vi "1.7A_Test.vi"(3 "error in":errorcluster) -> (10 "error out":errorcluster)   [LabVIEW 2015]
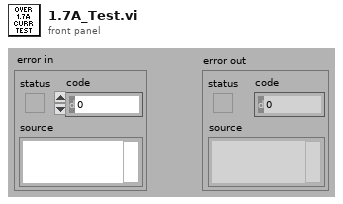
[diagram p1: front panel]
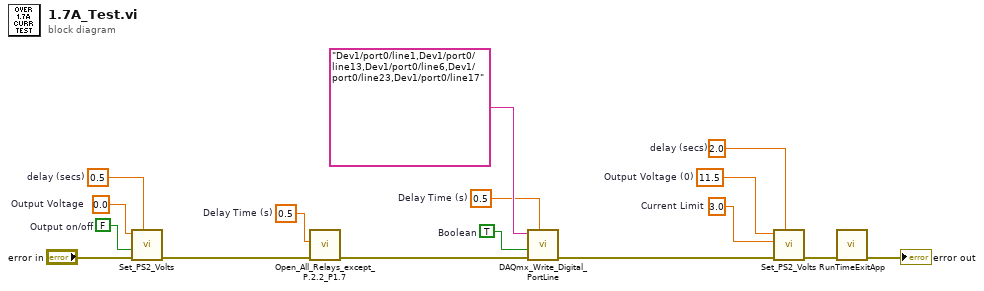
[diagram p0: block diagram]
diagram:
  w1 = 3.0  # Current Limit
  w2 = 0.5  # Delay Time (s)
  w3 = 0.5  # Delay Time (s)
  w6 = 0.0  # Output Voltage
  w7 = 0.5  # delay (secs)
  w8 = FALSE  # Output on/off
  w10 = 2.0  # delay (secs)
  w14 = 11.5  # Output Voltage (0)
  w16 = TRUE  # Boolean
  n1 = call "Set_PS2_Volts.vi"("delay (secs)"=w7, "error in"="error in", "Output on/off"=w8, "Output Voltage"=w6) -> ("error out"=w4:errorcluster)  [unwired: 5 in, 2 out]
  n2 = call "Open_All_Relays_except_P.2.2_P1.7.vi"("Delay Time (s)"=w3, "error in"=w4) -> ("error out"=w9:errorcluster)  [unwired: 7 in]
  n3 = call "DAQmx_Write_Digital_PortLine.vi"("Device/Ports/Lines"="Dev1/port0/line1,Dev1/port0/line13,Dev1/port0/line6,Dev1/port0/line23,Dev1/port0/line17", "Boolean"=w16, "error in"=w9, "Delay Time (s)"=w2) -> ("error out"=w13:errorcluster)  [unwired: 5 in, 1 out]
  n4 = call "Set_PS2_Volts.vi"("delay (secs)"=w10, "error in"=w13, "Current Limit"=w1, "Output Voltage"=w14) -> ("error out"=w11:errorcluster)  [unwired: 5 in, 2 out]
  n5 = call "RunTimeExitApp.vi"("error in (no error)"=w11) -> ("error out"=→"error out":errorcluster)  [unwired: 10 in]
